vi "timestamp millisec change in shift.vi"(10 "fractional second":dbl, 11 "time stamp in":timestamp) -> (3 "time stamp out":timestamp)   [LabVIEW 2017]
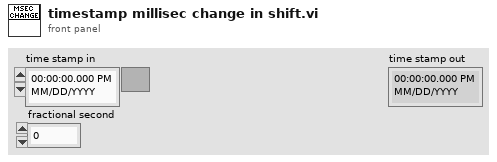
[diagram p1: front panel]
types:
  T1 = typedef "LVDateTimeRec.ctl" = cluster{"fractional second":dbl, "second":i32, "minute":i32, "hour":i32, "day of month":i32, "month":i32, "year":i32, "day of week":i32, "day of year":i32, "DST":i32}
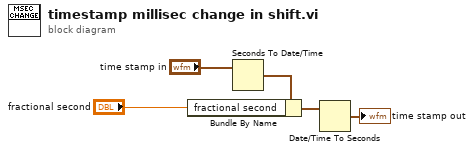
[diagram p0: block diagram]
diagram:
  n1 = Seconds To Date/Time(time stamp (now)="time stamp in") -> (date time rec=w4:T1)  [unwired: 1 in]
  n2 = Bundle By Name(cluster=w4, "fractional second"="fractional second") -> (w5:T1)
  n3 = Date/Time To Seconds(2:w5) -> (0:→"time stamp out":timestamp)  [unwired: 1 in]
